vi "run.vi"(8 "error in (no error)":errorcluster, 10 "Log in":refnum<class "Log.lvclass">, 11 "ICCameraController in":refnum<class "ICCameraController.lvclass">) -> (0 "error out":errorcluster, 2 "Log out":refnum<class "Log.lvclass">, 3 "ICCameraController out":refnum<class "ICCameraController.lvclass">)   [LabVIEW 2011, in "Hardware.lvlib" / "Channels.lvlib" / "ICCameraController.lvclass"]
uses:
  ICCameraController.lvclass
  Tools/Log.lvclass
  ICCameraController.lvclass/ICCameraController.ctl
  ICCameraAcquisitor/ICCameraAcquisitor.lvclass
panel:
  in  "ICImagingControl":refnum<k7>(container)
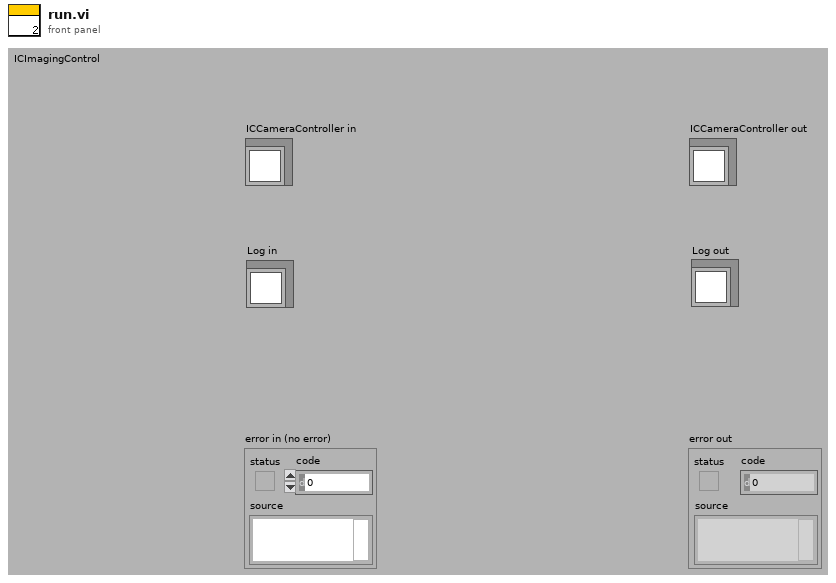
[diagram p1: front panel]
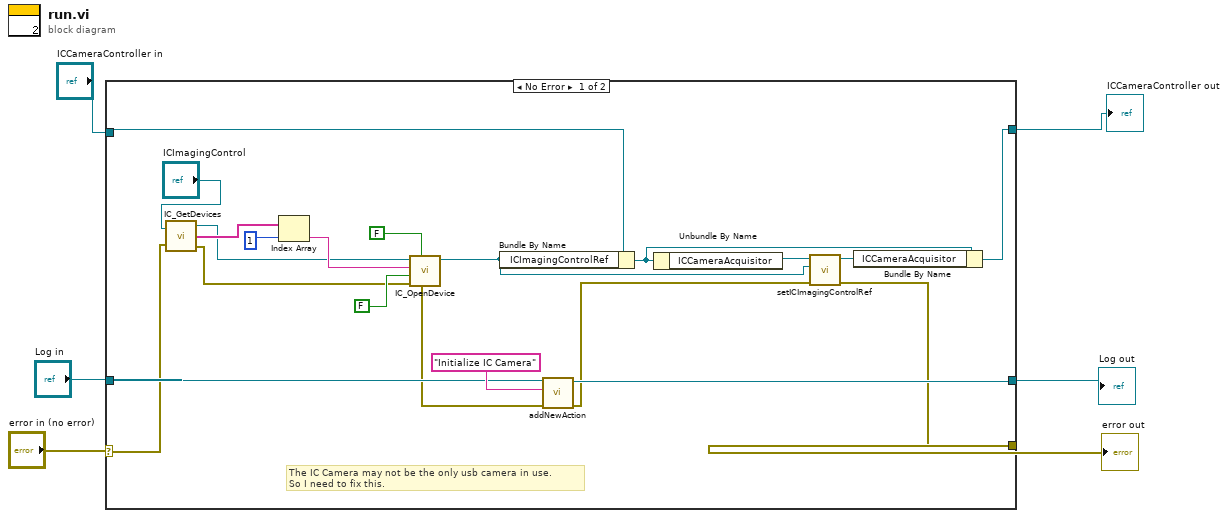
[diagram p0: block diagram]
diagram:
  n1 = case shown="No Error" "error in (no error)" {
    selector: "error in (no error)" -> [w19 w28]
    tunnel: "ICCameraController in" -> [w17 w30]
    tunnel: [w11 w30] -> w4
    tunnel: [w26 w29] -> w3
    tunnel: "Log in" -> [w25 w29]
    tunnel: [w13 w28] -> w1
    frame No Error {
      # "The IC Camera may not be the only usb camera in use.\nSo I need to fix this."
      n2 = call <userlib>:"IC_GetDevices.vi"("ICImagingControl In"="ICImagingControl", "Error In (no error)"=w19) -> ("ICImagingControl Out"=w8:refnum<k7>, "Devices"=w24:string[], "Error Out"=w20:errorcluster)
      n3 = Index Array(array=w24, index=1) -> (element=w23:string)
      n4 = call <userlib>:"IC_OpenDevice.vi"("Color"=FALSE, "Error In (no error)"=w20, "Live"=FALSE, "Device"=w23, "ICImagingControl In"=w8) -> ("ICImagingControl Out"=w15:refnum<k7>, "Error Out"=w18:errorcluster)  [unwired: 1 in, 4 out]
      n5 = Bundle By Name(cluster=w17, "ICImagingControlRef"=w15) -> (w12:refnum<class "ICCameraController.lvclass">)
      n6 = call-dynamic "addNewAction.vi"("error in (no error)"=w18, "newAction"="Initialize IC Camera", "Log in"=w25) -> ("error out"=w14:errorcluster, "Log out"=w26:refnum<class "Log.lvclass">)  [unwired: 7 in]
      n7 = Unbundle By Name(w12) -> ("ICCameraAcquisitor"=w16:refnum<class "ICCameraAcquisitor.lvclass">)
      n8 = call "setICImagingControlRef.vi"("error in (no error)"=w14, "ICImagingControlRef"=w15, "ICCameraAcquisitor.lvclass in"=w16) -> ("error out"=w13:errorcluster, "ICCameraAcquisitor.lvclass out"=w10:refnum<class "ICCameraAcquisitor.lvclass">)  [unwired: 7 in]
      n9 = Bundle By Name(cluster=w12, "ICCameraAcquisitor"=w10) -> (w11:refnum<class "ICCameraController.lvclass">)
    }
    frame Error {
    }
  }
  "error out" <- w1
  "ICCameraController out" <- w4
  "Log out" <- w3
